vi "Menu.Filter.vi"(8 "error in (no error)":errorcluster, 10 "state variables in":T4, 11 "Menu in":refnum<k9>) -> (0 "error out":errorcluster)   [LabVIEW 2015, in "Multihead GUI.lvlib"]
uses:
  Multihead GUI.lvlib
  <vilib>/NI Veristand/Execution/Workspace/WorkspaceAPI.ctl
  NationalInstruments.VeriStand.ClientAPI
  <vilib>/NI Veristand/Execution/Workspace/SystemStateEventRef.ctl
  <vilib>/NI Veristand/Execution/Workspace/Target State Info.ctl
  <vilib>/NI Veristand/Execution/Workspace/Target State.ctl
  <vilib>/NI Veristand/Execution/Workspace/SystemStateRegEventRef.ctl
  Execution GUI/SubVIs/Main.Constants.vi
  Execution GUI/Single Station Execution.lvlib
  Shared/Shared.lvlib
  <vilib>/NI Veristand/Execution/Workspace/NI_VS Workspace ExecutionAPI.lvlib
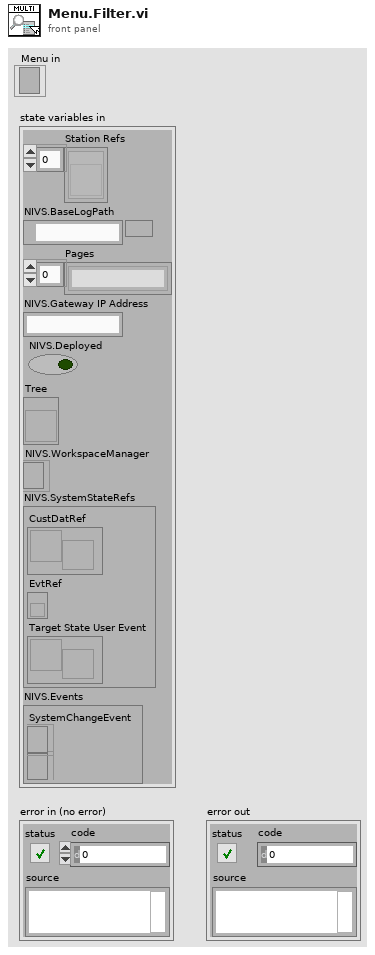
[diagram p1: front panel]
types:
  T1 = typedef "NI_VS Workspace ExecutionAPI.lvlib/WorkspaceAPI.ctl" = refnum<k24>
  T2 = typedef "NI_VS Workspace ExecutionAPI.lvlib/SystemStateEventRef.ctl" = cluster{"CustDatRef":refnum<user-event>, "EvtRef":refnum<k27>, "Target State User Event":refnum<user-event>}
  T3 = typedef "NI_VS Workspace ExecutionAPI.lvlib/SystemStateRegEventRef.ctl" = refnum<event-registration>
  T4 = cluster{"Station Refs":refnum<vi>[], "NIVS.BaseLogPath":path, "Pages":string[], "NIVS.Gateway IP Address":string, "NIVS.Deployed":bool, "Tree":refnum<vi>, "NIVS.WorkspaceManager":T1, "NIVS.SystemStateRefs":T2, "NIVS.Events":cluster{"SystemChangeEvent":T3, "WorkspaceEvent":refnum<event-registration>}}
  T5 = typedef "Single Station Execution.lvlib/Stimulus.Status.ctl" = cluster{"Restart":bool, "NIVS.SequenceState":T6, "Alarmed?":bool, "Disable?":bool}
  T6 = typedef "Single Station Execution.lvlib/Execution.SequenceState.ctl" = enum16{"Idle", "Initializing", "Running", "Paused", "Finalizing", "Complete"}
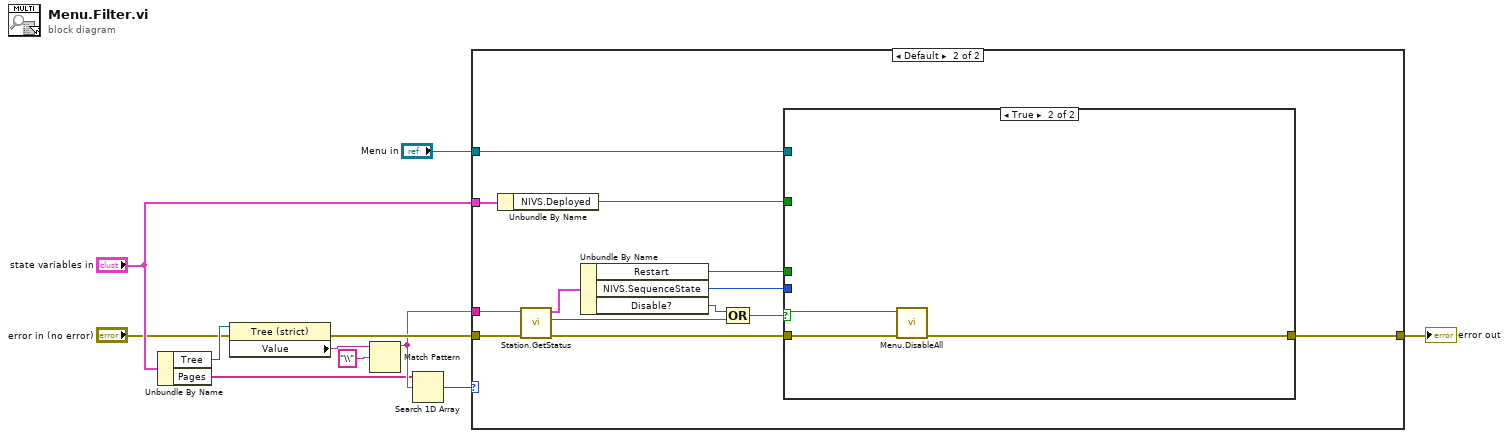
[diagram p0: block diagram]
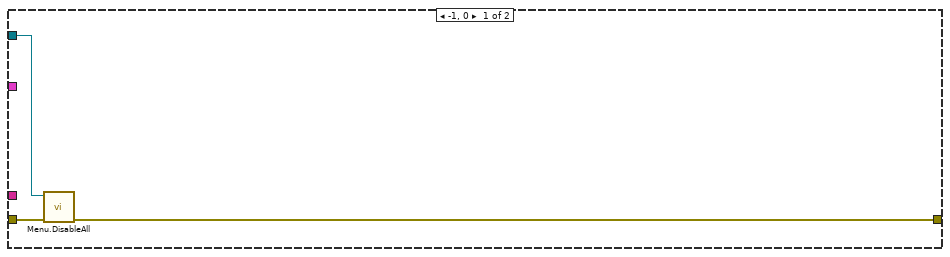
[diagram p2: hidden frame]
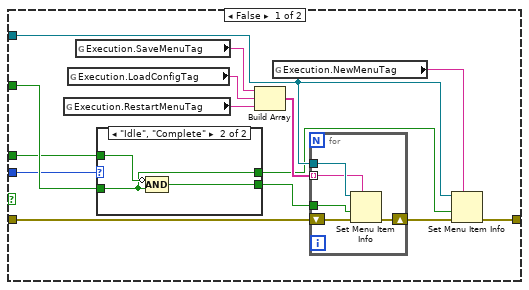
[diagram p3: hidden frame]
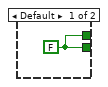
[diagram p4: hidden frame]
diagram:
  n1 = Unbundle By Name("state variables in") -> ("Tree"=w8:refnum<vi>, "Pages"=w1:string[])
  n2 = property class="Tree (strict)"(reference=w8, error in="error in (no error)") -> (error out=w10:errorcluster, "Value"=w2:string)  [unwired: 1 out]
  n3 = Match Pattern(string=w2, regular expression="\\") -> (before substring=w4:string)  [unwired: 1 in, 3 out]
  n4 = Search 1D Array(1D array=w1, element=w4) -> (index of element=w5:i32)  [unwired: 1 in]
  n5 = case shown="Default" w5 {
    tunnel: w4 -> [_ w23]
    tunnel: "state variables in" -> [_ w26]
    tunnel: "Menu in" -> [w14 w25]
    tunnel: w10 -> [w13 w22]
    tunnel: [w12 w24] -> w11
    frame -1, 0 {
      n6 = call "Menu.DisableAll.vi"("error in (no error)"=w13, "Menu in"=w14) -> ("error out"=w12:errorcluster)  [unwired: 9 in]
    }
    frame Default {
      n7 = Unbundle By Name(w26) -> ("NIVS.Deployed"=w27:bool)
      n8 = call "Station.GetStatus.vi"("error in (no error)"=w22, "Station.ID"=w23) -> ("error out"=w21:errorcluster, "timed out?"=w16:bool, "Station.Status"=w20:T5)  [unwired: 7 in]
      n9 = Unbundle By Name(w20) -> ("Restart"=w19:bool, "NIVS.SequenceState"=w18:T6, "Disable?"=w17:bool)
      n10 = Compound Arithmetic op=OR(w17, w16) -> (w15:bool)
      n11 = case shown="True" w15 {
        tunnel: w27 -> [w40 _]
        tunnel: w25 -> [w35 w51]
        tunnel: [w31 w52] -> w24
        tunnel: w21 -> [w30 w53]
        tunnel: w19 -> [w29 _]
        tunnel: w18 -> [w28 _]
        frame False {
          n12 = global read "Main.Constants.vi" "Execution.RestartMenuTag"() -> (w41:string)
          n13 = global read "Main.Constants.vi" "Execution.LoadConfigTag"() -> (w37:string)
          n14 = global read "Main.Constants.vi" "Execution.SaveMenuTag"() -> (w32:string)
          n15 = case shown="\"Idle\", \"Complete\"" w28 {
            tunnel: [w47 w50] -> w38
            tunnel: w40 -> [_ w48]
            tunnel: w29 -> [_ w49]
            tunnel: [w47 w48] -> w34
            frame Default {
              w47 = FALSE
            }
            frame "Idle", "Complete" {
              n16 = Compound Arithmetic op=AND(invert w49, w48) -> (w50:bool)
            }
          }
          n17 = Build Array(w32, w37, w41) -> (w39:string[])
          n18 = global read "Main.Constants.vi" "Execution.NewMenuTag"() -> (w33:string)
          n19 = for {
            tunnel: w35 -> [w46]
            tunnel: w38 -> [w45]
            tunnel: w39 -> [w44] mode=indexing
            shift-right: [w42] -> w36
            shift-left: w30 -> [w43]
            n20 = Set Menu Item Info(7:w44, 8:w43, 9:w45, 11:w46) -> (0:w42:errorcluster)  [unwired: 3 in, 1 out]
          }
          n21 = Set Menu Item Info(7:w33, 8:w36, 9:w34, 11:w35) -> (0:w31:errorcluster)  [unwired: 3 in, 1 out]
        }
        frame True {
          n22 = call "Menu.DisableAll.vi"("error in (no error)"=w53, "Menu in"=w51) -> ("error out"=w52:errorcluster)  [unwired: 9 in]
        }
      }
    }
  }
  "error out" <- w11
